vi "Configure Waveform.vi"(4 "Phase Unit (0: Radian)":u16(ring) items=["Radians", "Degrees"], 5 "Frequency (1000 Hz)":dbl=1000.0, 6 "Phase (0)":dbl, 7 "DC Offset (0.00 V)":dbl, 8 "error in (no error)":errorcluster, 9 "Amplitude (1 Vpp)":dbl=1.0, 10 "Channel (1 Channel 1)":u16(ring)=1 items=["Channel 1"=1, "Channel 2"=2], 11 "VISA resource name":refnum<visa-resource-name>) -> (0 "error out":errorcluster, 3 "VISA resource name out":refnum<visa-resource-name>)   [LabVIEW 2016, in "Tektronix AFG 1000 Series.lvlib"]
doc: "Selects the frequency, amplitude, offset, and phase for a standard waveform or arbitrary waveform."
uses:
  Tektronix AFG 1000 Series.lvlib
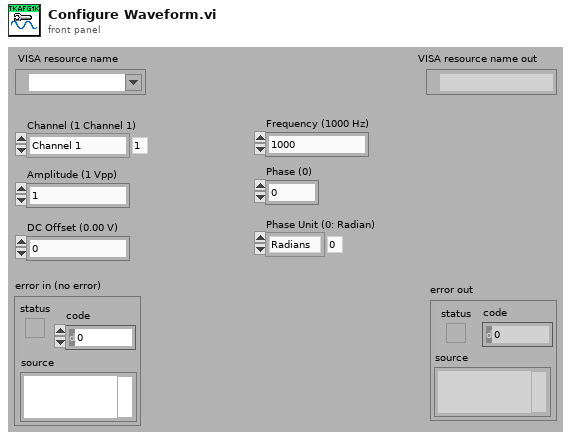
[diagram p1: front panel]
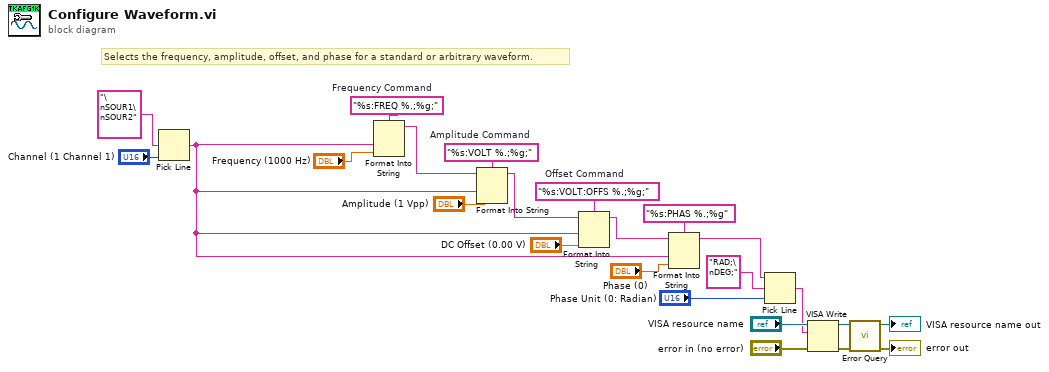
[diagram p0: block diagram]
diagram:
  w16 = "%s:VOLT:OFFS %.;%g;"  # Offset Command
  w17 = "%s:VOLT %.;%g;"  # Amplitude Command
  w18 = "%s:FREQ %.;%g;"  # Frequency Command
  # "Selects the frequency, amplitude, offset, and phase for a standard or arbitrary waveform."
  n1 = Pick Line(multi-line string="\nSOUR1\nSOUR2" ("string (\"\")"), line index="Channel (1 Channel 1)") -> (output string=w5:string)  [unwired: 1 in]
  n2 = Format Into String(format string=w18, w5, "Frequency (1000 Hz)") -> (resulting string=w14:string)  [unwired: 2 in, 1 out]
  n3 = Format Into String(format string=w17, initial string=w14, w5, "Amplitude (1 Vpp)") -> (resulting string=w15:string)  [unwired: 1 in, 1 out]
  n4 = Format Into String(format string=w16, initial string=w15, w5, "DC Offset (0.00 V)") -> (resulting string=w7:string)  [unwired: 1 in, 1 out]
  n5 = Format Into String(format string="%s:PHAS %.;%g", initial string=w7, w5, "Phase (0)") -> (resulting string=w3:string)  [unwired: 1 in, 1 out]
  n6 = Pick Line(string ("")=w3, multi-line string="RAD;\nDEG;", line index="Phase Unit (0: Radian)") -> (output string=w1:string)
  n7 = VISA Write(VISA resource name="VISA resource name", write buffer=w1, error in (no error)="error in (no error)") -> (VISA resource name out=w20:refnum<visa-resource-name>, error out=w19:errorcluster)  [unwired: 1 out]
  n8 = call "Error Query.vi"("error in (no error)"=w19, "VISA resource name"=w20) -> ("error out"=→"error out":errorcluster, "VISA resource name out"=→"VISA resource name out":refnum<visa-resource-name>)  [unwired: 6 in, 2 out]
